vi "OpenCVCam_ClassCast.vi"(11 "OpenCVCam in":refnum<class>) -> (3 "OpenCVCam out":refnum<class "OpenCVCam.lvclass">)   [LabVIEW 2021, in "OpenCVCam.lvclass"]
uses:
  OpenCVCam.lvclass
  OpenCVCam.lvclass/OpenCVCam.ctl
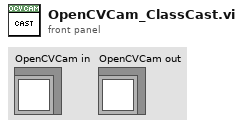
[diagram p1: front panel]
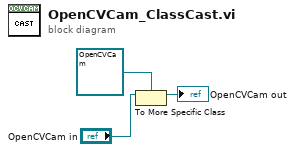
[diagram p0: block diagram]
diagram:
  n1 = To More Specific Class(target class=refnum<class "OpenCVCam.lvclass"> refnum ("reference in"), reference="OpenCVCam in") -> (specific class reference=→"OpenCVCam out":refnum<class "OpenCVCam.lvclass">)  [unwired: 1 in, 1 out]
